vi "DQMH Tester Prepare hse-appl - Get Name and Path.vi"(8 "error in":errorcluster, 11 "Real-Time App Name":string) -> (0 "error out":errorcluster, 2 "Project Path":path, 3 "Project Name":string)   [LabVIEW 2014, in "hse-dqmh.lvlib"]
uses:
  hse-dqmh.lvlib
  <vilib>/regexp/Match Regular Expression.xnode
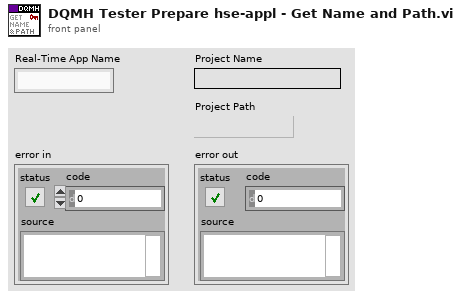
[diagram p1: front panel]
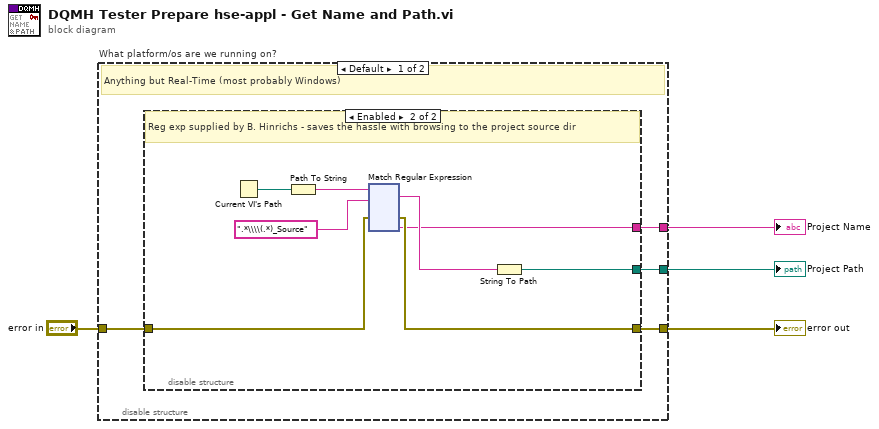
[diagram p0: block diagram]
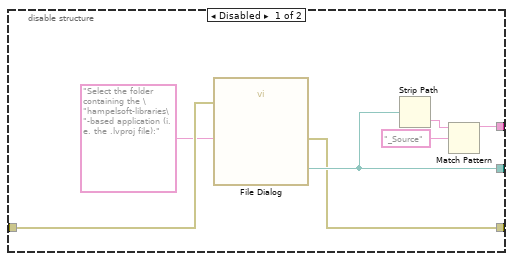
[diagram p2: hidden frame]
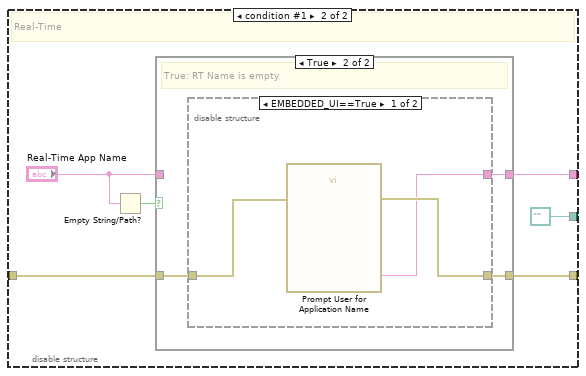
[diagram p3: hidden frame]
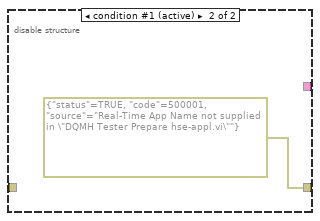
[diagram p5: hidden frame]
diagram:
  n1 = disable-structure "What platform/os are we running on?" shown="Default" {
    disable-tunnel: [w8 path "" ("selected path")] -> w2
    disable-tunnel: [w7 w144] -> w3
    disable-tunnel: [w6 w145] -> w4
    disable-tunnel: "error in" -> [w5 w141]
    frame condition #0 (active) {
      # "Anything but Real-Time (most probably Windows)"
      n2 = disable-structure shown="Enabled" {
        disable-tunnel: [w15 w17] -> w8
        disable-tunnel: [w12 w18] -> w7
        disable-tunnel: [w11 w23] -> w6
        disable-tunnel: w5 -> [w10 w16]
        frame Disabled {
          n3 = call "File Dialog"("prompt"="Select the folder containing the \"hampelsoft-libraries\"-based application (i.e. the .lvproj file):", "error in"=w10) -> ("selected path"=w15:path, "error out"=w11:errorcluster)  [unwired: 10 in, 2 out]
          n4 = Strip Path(path=w15) -> (name=w14:string)  [unwired: 1 out]
          n5 = Match Pattern(string=w14, regular expression="_Source") -> (before substring=w12:string)  [unwired: 1 in, 3 out]
        }
        frame Enabled {
          # "Reg exp supplied by B. Hinrichs - saves the hassle with browsing to the project source dir"
          n6 = Current VI's Path() -> (path=w22:path)
          n7 = Path To String(path=w22) -> (string=w21:string)
          n8 = xnode "Match Regular Expression"("input string"=w21, "regular expression"=".*\\\\(.*)_Source", "error in"=w16) -> ("whole match"=w20:string, "error out"=w23:errorcluster, "submatch 1"=w18:string)  [unwired: 3 in, 3 out]
          n9 = String To Path(string=w20) -> (path=w17:path)
        }
      }
    }
    frame condition #1 {
      # "Real-Time"
      n10 = Empty String/Path?(string/path="Real-Time App Name") -> (empty?=w142:bool)
      n11 = case shown="True" w142 {
        tunnel: [w147 w150] -> w145
        tunnel: [w146 w149] -> w144
        tunnel: w141 -> [w147 w148]
        tunnel: "Real-Time App Name" -> [w146 _]
        frame False {
          # "False: RT Name not empty"
        }
        frame True {
          # "True: RT Name is empty"
          n12 = disable-structure shown="EMBEDDED_UI==True" {
            disable-tunnel: [w153 errorcluster {"status"=TRUE, "code"=500001, "source"="Real-Time App Name not supplied in \"DQMH Tester Prepare hse-appl.vi\""} ("error out")] -> w150
            disable-tunnel: [w152 _] -> w149
            disable-tunnel: w148 -> [w151 _]
            frame condition #0 {
              n13 = call "Prompt User for Application Name"("error in (no error)"=w151) -> ("Application Name"=w152:string, "error out"=w153:errorcluster)  [unwired: 16 in, 1 out]
            }
            frame condition #1 (active) {
            }
          }
        }
      }
    }
  }
  "error out" <- w4
  "Project Name" <- w3
  "Project Path" <- w2
